vi "tt20_make_histo_plot.vi"(8 "error in (no error)":errorcluster, 10 "panel in":refnum<class "panel.lvclass">, 11 "tt20 in":refnum<class "tt20.lvclass">) -> (0 "error out":errorcluster, 2 "panel out":refnum<class "panel.lvclass">, 3 "tt20 out":refnum<class "tt20.lvclass">)   [LabVIEW 2015, in "tt20.lvclass"]
uses:
  tt20.lvclass
  UI/panel_class/panel.lvclass
  UI/panel_class/panel.lvclass/panel.ctl
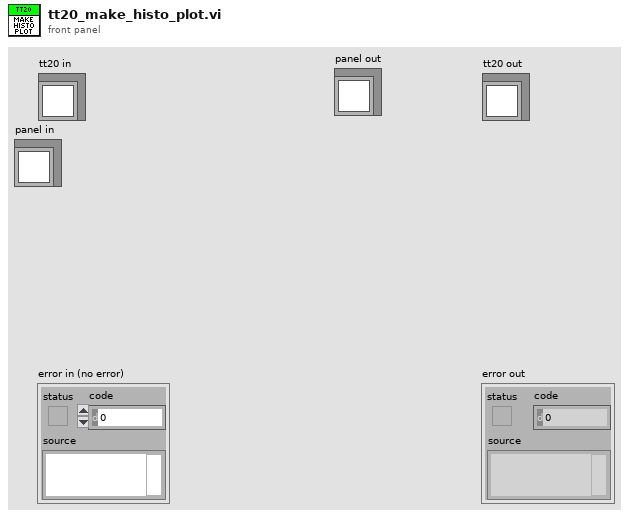
[diagram p1: front panel]
types:
  T1 = enum32{"Chart", "Graph", "Map", "XY Graph", "Large Readout"}
  T2 = typedef "ui_plot_references.ctl" = cluster{"plots":refnum<vi>, "chart":refnum<vi>, "graph":refnum<vi>, "map":refnum<vi>, "XY Graph":refnum<vi>}
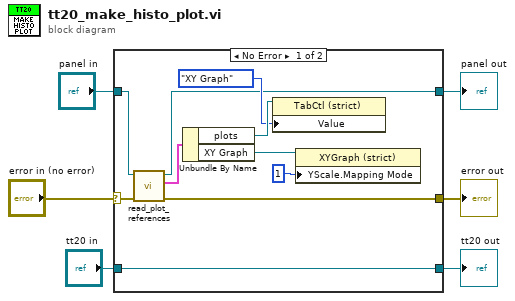
[diagram p0: block diagram]
diagram:
  n1 = case shown="No Error" "error in (no error)" {
    selector: "error in (no error)" -> [w13 w19]
    tunnel: [w10 w19] -> w5
    tunnel: [w14 w18] -> w3
    tunnel: "tt20 in" -> [w14 w18]
    tunnel: "panel in" -> [w16 w17]
    tunnel: [w9 w17] -> w1
    frame No Error {
      n2 = call "read_plot_references.vi"("error in (no error)"=w13, "panel in"=w16) -> ("error out"=w10:errorcluster, "plot_references"=w15:T2, "panel out"=w9:refnum<class "panel.lvclass">)  [unwired: 7 in]
      n3 = Unbundle By Name(w15) -> ("plots"=w12:refnum<vi>, "XY Graph"=w7:refnum<vi>)
      n4 = property class="TabCtl (strict)"(reference=w12, "Value"=T1."XY Graph") -> ()  [unwired: 1 in, 2 out]
      n5 = property class="XYGraph (strict)"(reference=w7, "YScale.Mapping Mode"=u8 1 ("Y Scale.Mapping Mode")) -> ()  [unwired: 1 in, 2 out]
    }
    frame Error {
    }
  }
  "error out" <- w5
  "tt20 out" <- w3
  "panel out" <- w1
